vi "Exec Macro.vi"(8 "error in (no error)":errorcluster, 9 "Array of States LUT":variant[](array[variant]), 10 "States LUT (name -> boolean state)":variant, 11 "Motions in":refnum<class "Motions.lvclass">) -> (0 "error out":errorcluster, 3 "Motions out":refnum<class "Motions.lvclass">)   [LabVIEW 2016, in "Hardware.lvlib" / "Motions.lvlib" / "Motions.lvclass"]
uses:
  <userlib>/Common Components/Hardware/Abstract System/Motions/Motions/Motions.lvclass
  <userlib>/Common Components/Hardware/Abstract System/Motions/Motions/Motions.lvclass/Motions.ctl
  <userlib>/Common Components/TriggerAction Q/TriggerAction Q/TriggerAction Q.lvclass/TriggerAction Q.ctl
  <userlib>/Common Components/TriggerAction Q/TriggerAction Q/Run (hybrid).vi
  <userlib>/Common Components/TriggerAction Q/TriggerAction Q/TriggerAction Q.lvclass
panel:
  # "System level states"
  # "States of each motion"
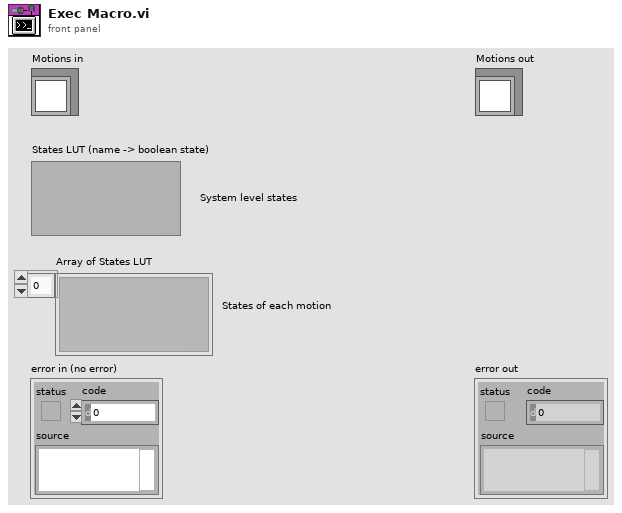
[diagram p1: front panel]
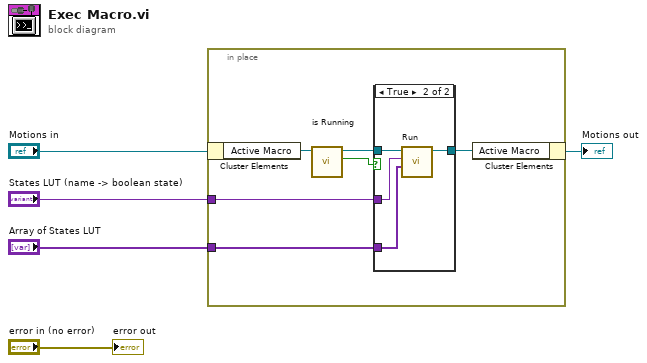
[diagram p0: block diagram]
diagram:
  n1 = in-place {
    in-place-border: "Array of States LUT" -> [w7]
    in-place-border: "States LUT (name -> boolean state)" -> [w6]
    n2 = in-place-cluster #1("Motions in") -> ("Active Macro"=w10:refnum<class "TriggerAction Q.lvclass">)
    n3 = call <userlib>:"is Running.vi"("TriggerAction in"=w10) -> ("Running?"=w8:bool, "TriggerAction out"=w11:refnum<class "TriggerAction Q.lvclass">)  [unwired: 9 in]
    n4 = case shown="True" w8 {
      tunnel: w11 -> [w12 w16]
      tunnel: [w12 w15] -> w9
      tunnel: w7 -> [_ w14]
      tunnel: w6 -> [_ w13]
      frame False {
      }
      frame True {
        n5 = call-poly <userlib>:"Run.vi"("Array of States LUT"=w14, "States LUT (name -> boolean state)"=w13, "TriggerAction in"=w16) -> ("TriggerAction out"=w15:refnum<class "TriggerAction Q.lvclass">)  [unwired: 7 in, 1 out]
      }
    }
    n6 = in-place-cluster #1("Active Macro"=w9) -> (→"Motions out":refnum<class "Motions.lvclass">)
  }
  "error out" <- "error in (no error)"
